vi "Read Depth.vi"(8 "error in (no error)":errorcluster) -> (0 "error out":errorcluster, 3 "Depth image":picture)   [LabVIEW 2017]
uses:
  libkinect_wrapper.dll
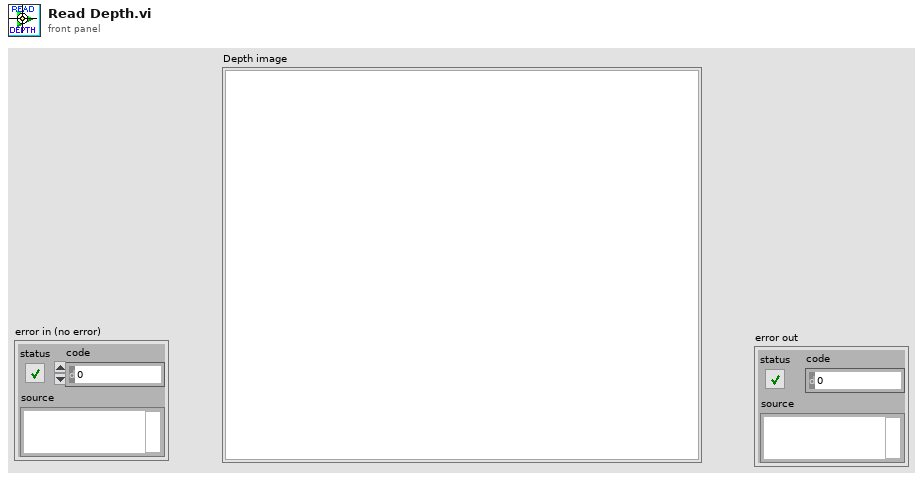
[diagram p1: front panel]
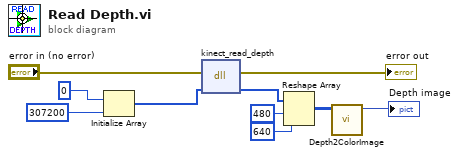
[diagram p0: block diagram]
diagram:
  n1 = Initialize Array(u16 0 ("element"), 307200) -> (w10:u16[])
  n2 = dll-call lib="libkinect_wrapper.*" fn="kinect_read_depth"(error in="error in (no error)", "depth"=w10) -> (error out=→"error out":errorcluster, "depth"=w5:u16[])  [unwired: 3 in, 1 out]
  n3 = Reshape Array(w5, 480 ("dimension size"), 640 ("dimension size")) -> (w1:u16[][])
  n4 = call "Depth2ColorImage.vi"("Depth"=w1) -> ("HSV Image"=→"Depth image":picture)  [unwired: 10 in]
